vi "FugacityGraphWithTablesLowT.vi"(1 "Fugacity table":dbl[](array[numeric])=[0.0, 0.0], 2 "Temperature table":dbl[](array[numeric])=[0.0, 0.0]) -> (0 "Array":cluster{"Array":dbl[], "Array 2":dbl[]}[](array[cluster]))   [LabVIEW 2009]
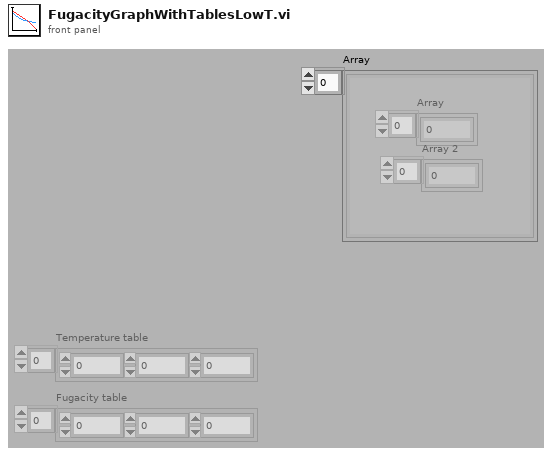
[diagram p1: front panel]
types:
  T1 = cluster{"Temperature table":dbl[], "Fugacity table":dbl[]}
  T2 = cluster{"Temperature table":dbl[], "Fugacity table":dbl[]}[]
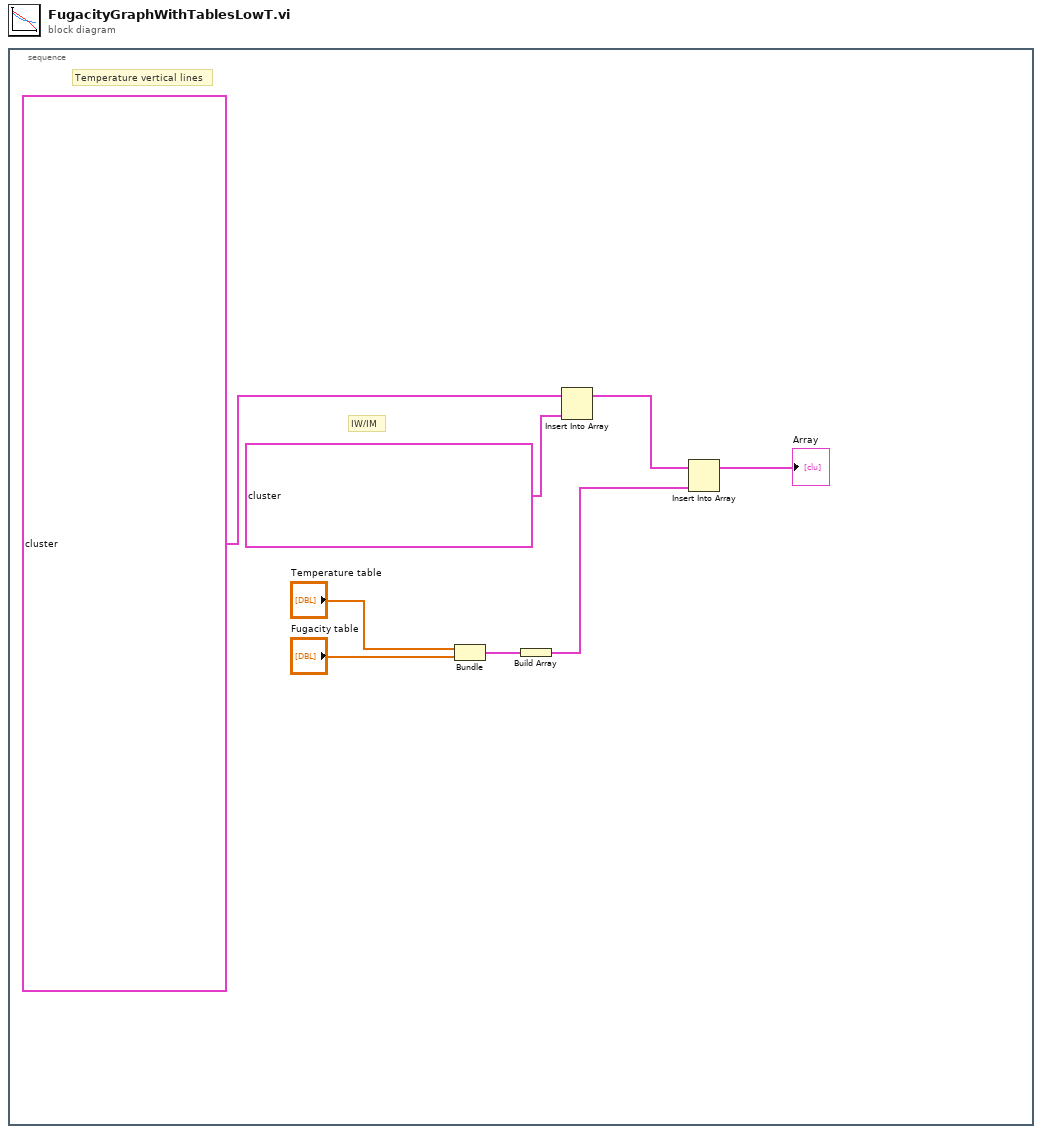
[diagram p0: block diagram]
diagram:
  n1 = stacked-sequence {
    frame #0 {
      # "IW/IM"
      # "Temperature vertical lines"
      n2 = Bundle("Temperature table"="Temperature table", "Fugacity table"="Fugacity table") -> (w4:T1)  [unwired: 1 in]
      n3 = Build Array(w4) -> (w5:T2)
      n4 = Insert Into Array(array=cluster{ext[], ext[]}[] [{[17.44743958824043, 17.44743958824043], [-15.0, -90.0]}, {[14.85552997103172, 14.85552997103172], [-15.0, -90.0]}, {[12.93410075664489, 12.93410075664489], [-15.0, -90.0]}, {[11.45278589016778, 11.45278589016778], [-15.0, -90.0]}, {[10.2759081333812900003, 10.2759081333812900003], [-15.0, -90.0]}, {[9.318361831989936, 9.318361831989936], [-15.0, -90.0]}, {[21.129999999999999999, 21.129999999999999999], [-15.0, -90.0]}, {[26.8, 26.8], [-15.0, -90.0]}, {[33.650000000000000001, 33.650000000000000001], [-15.0, -90.0]}], new element=cluster{ext[], ext[]}[] [{[9.0, 11.83374083129584, 33.650000000000000001, 33.650000000000000001], [-17.9235, -25.63552567237164, -89.480000000000000003, -89.480000000000000003]}]) -> (w6:cluster{ext[], ext[]}[])  [unwired: 1 in]
      n5 = Insert Into Array(array=w6, new element=w5) -> (→"Array":cluster{ext[], ext[]}[])  [unwired: 1 in]
    }
  }
